vi "nanocal -- nuclear schottky fit V4.vi"() -> ()   [LabVIEW 2020] (continued)
"IDS0323_210901_RAW_cal_CeCoIn5_4th_052(138)_C(f)_12T_3.10K_45deg_Tdep_raw_.dat", "IDS0372_210908_RAW_cal_CeCoIn5_4th_102_C(f)_12.0T_3.11K_60deg_Tdep_raw_.dat", "IDS0393_210910_RAW_cal_CeCoIn5_4th_123_C(f)_8.0T_3.11K_0deg_Tdep_raw_.dat", "IDS0171_210310_RAW_cal_CeCoIn5_2nd_060_12T_fsweep_3.19K_0deg_Tdep_raw_.dat", "IDS0196_210310_RAW_cal_CeCoIn5_2nd_084_12T_5.7K_90deg_Tdep_raw_.dat", "IDS0324_210901_RAW_cal_CeCoIn5_4th_053(139)_C(f)_12T_5.70K_45deg_Tdep_raw_.dat", "IDS0373_210908_RAW_cal_CeCoIn5_4th_103_C(f)_12.0T_5.75K_60deg_Tdep_raw_.dat", "IDS0394_210910_RAW_cal_CeCoIn5_4th_124_C(f)_8.0T_5.75K_0deg_Tdep_raw_.dat", "IDS0172_210310_RAW_cal_CeCoIn5_2nd_061_12T_fsweep_5.8K_0deg_Tdep_raw_.dat"]
  in  "generate empty string from filelist !":bool
  in  "toggle generate labview files":bool
  in  "data file formatting":T13=enum."raw nanocal"
  in  "side":T14=enum."ref"
  in  "string notes":string="\"T\"-> 0.225000,    \"ζ\"-> 0.006057  , \"τ1\"-> 0.011106  , \"τS\"-> 0.134857  , \"τN\"-> 0.000042  , \"τC\"-> 0.012982  , \"κ0\"-> 0.000000101776  , \"mm1\"-> 0.000071  , \"mm2\"-> 0.148631  , \"mm3\"-> 0.011103 "
  in  "load! :l":bool
  in  "Read from file":path=path "/opt/new/Dropbox/shared_AkashAndreas/paper-CeCoIn5/Original RAW data/Original RAW files (IDS0272 to IDS03xx)/IDS0340_210904_RAW_cal_CeCoIn5_4th_069_C(f)_5.0T_0.308K_90deg_Tdep_raw_.dat"
  in  "parse! :p":bool
  in  "String":string=" <| \"ζ\"->  0.269210160049  , \"τ1\"-> 0.027533256233  , \"τS\"-> 0.109874895668  , \"τN\"-> 0.015552411517  , \"τC\"-> 0.001074349295  , \"κ0\"-> 0.000000000732  , \"mm1\"-> 0.000000000000  , \"mm2\"-> 0.000000000000  , \"mm3\"-> 0.000000000000  , \"T\"->  0.308000000000  , \"B\"-> 5.000000000000  , \"θ\"-> 90.000000000000  |> "
  out "notes":string="------------\n\n/opt/new/Dropbox/desktop_data/Indium-nanocal-cell12-June2021/labview-ready-files\nIndium_June2021_*_ark.dat\n\n---------------------\n/opt/new/Dropbox/shared_AkashAndreas/paper-CeCoIn5/labviewreadydata\nCeCoIn5_*_labview_.dat\n--------------------------------\n\n  48 ->   <| \"ζ\"->  0.219100303741  , \"τ1\"-> 0.028643012604  , \"τS\"-> 0.279362928811  , \"τN\"-> 0.246156444058  , \"τC\"-> 0.001272401549  , \"κ0\"-> 0.000000000760  , \"mm1\"-> 0.000227975653  , \"mm2\"-> 0.014929571562  , \"mm3\"-> 0.655418694024  , \"T\"->  0.148000000000  , \"B\"-> 12.000000000000  , \"θ\"-> 0.000000000000  |>   , \r49 ->   <| \"ζ\"->  0.172530402516  , \"τ1\"-> 0.028151242536  , \"τS\"-> 0.147833386881  , \"τN\"-> 0.151615465647  , \"τC\"-> 0.001078987959  , \"κ0\"-> 0.000000001040  , \"mm1\"-> 0.000157922197  , \"mm2\"-> 0.013374167913  , \"mm3\"-> 0.366811023972  , \"T\"->  0.179000000000  , \"B\"-> 12.000000000000  , \"θ\"-> 0.000000000000  |>   , \r50 ->   <| \"ζ\"->  0.133463068512  , \"τ1\"-> 0.025720252342  , \"τS\"-> 0.123146502099  , \"τN\"-> 0.097478248186  , \"τC\"-> 0.001335222055  , \"κ0\"-> 0.000000001204  , \"mm1\"-> 0.000155896243  , \"mm2\"-> 0.013755191011  , \"mm3\"-> 0.263214393590  , \"T\"->  0.197000000000  , \"B\"-> 12.000000000000  , \"θ\"-> 0.000000000000  |>   , \r51 ->   <| \"ζ\"->  0.081993362741  , \"τ1\"-> 0.028064095915  , \"τS\"-> 0.091433392476  , \"τN\"-> 0.030443971714  , \"τC\"-> 0.001450504959  , \"κ0\"-> 0.000000001536  , \"mm1\"-> 0.000108446090  , \"mm2\"-> 0.019905820843  , \"mm3\"-> 0.141370833064  , \"T\"->  0.250000000000  , \"B\"-> 12.000000000000  , \"θ\"-> 0.000000000000  |>   , \r52 ->   <| \"ζ\"->  0.054088186012  , \"τ1\"-> 0.023838802615  , \"τS\"-> 0.069079396629  , \"τN\"-> 0.016435267456  , \"τC\"-> 0.002025071743  , \"κ0\"-> 0.000000001955  , \"mm1\"-> 0.000101234646  , \"mm2\"-> 0.018244822177  , \"mm3\"-> 0.097657814678  , \"T\"->  0.300000000000  , \"B\"-> 12.000000000000  , \"θ\"-> 0.000000000000  |>   , \r53 ->   <| \"ζ\"->  0.039314966212  , \"τ1\"-> 0.020712803909  , \"τS\"-> 0.055413767550  , \"τN\"-> 0.008474403424  , \"τC\"-> 0.002674063387  , \"κ0\"-> 0.000000002415  , \"mm1\"-> 0.000096818147  , \"mm2\"-> 0.017190811405  , \"mm3\"-> 0.072499170001  , \"T\"->  0.360000000000  , \"B\"-> 12.000000000000  , \"θ\"-> 0.000000000000  |>   , \r54 ->   <| \"ζ\"->  0.031945976845  , \"τ1\"-> 0.019000922826  , \"τS\"-> 0.045624146388  , \"τN\"-> 0.005314716063  , \"τC\"-> 0.002488383471  , \"κ0\"-> 0.000000002954  , \"mm1\"-> 0.000073272643  , \"mm2\"-> 0.016306894362  , \"mm3\"-> 0.057675293464  , \"T\"->  0.430000000000  , \"B\"-> 12.000000000000  , \"θ\"-> 0.000000000000  |>   , \r55 ->   <| \"ζ\"->  0.023031239946  , \"τ1\"-> 0.018268814012  , \"τS\"-> 0.037269400776  , \"τN\"-> 0.002696792890  , \"τC\"-> 0.003257395394  , \"κ0\"-> 0.000000003720  , \"mm1\"-> 0.000067670174  , \"mm2\"-> 0.016445281937  , \"mm3\"-> 0.045899921957  , \"T\"->  0.512000000000  , \"B\"-> 12.000000000000  , \"θ\"-> 0.000000000000  |>   , \r56 ->   <| \"ζ\"->  0.019920170845  , \"τ1\"-> 0.016368892412  , \"τS\"-> 0.030579536580  , \"τN\"-> 0.001736017565  , \"τC\"-> 0.004971418152  , \"κ0\"-> 0.000000004410  , \"mm1\"-> 0.000083939556  , \"mm2\"-> 0.015095997595  , \"mm3\"-> 0.039119658918  , \"T\"->  0.610000000000  , \"B\"-> 12.000000000000  , \"θ\"-> 0.000000000000  |>   , \r57 ->   <| \"ζ\"->  0.017558473054  , \"τ1\"-> 0.014545104284  , \"τS\"-> 0.022979681288  , \"τN\"-> 0.000840829385  , \"τC\"-> 0.005228030240  , \"κ0\"-> 0.000000006068  , \"mm1\"-> 0.000073916527  , \"mm2\"-> 0.013750428362  , \"mm3\"-> 0.030187552103  , \"T\"->  0.810000000000  , \"B\"-> 12.000000000000  , \"θ\"-> 0.000000000000  |>   , \r58 ->   <| \"ζ\"->  0.011916480594  , \"τ1\"-> 0.012551282481  , \"τS\"-> 0.018233218660  , \"τN\"-> 0.000345702746  , \"τC\"-> 0.004699451527  , \"κ0\"-> 0.000000008451  , \"mm1\"-> 0.000044190864  , \"mm2\"-> 0.012162820727  , \"mm3\"-> 0.023844039179  , \"T\"->  1.120000000000  , \"B\"-> 12.000000000000  , \"θ\"-> 0.000000000000  |>   , \r59 ->   <| \"ζ\"->  0.012831327568  , \"τ1\"-> 0.013315909415  , \"τS\"-> 0.012590836847  , \"τN\"-> 0.000065003013  , \"τC\"-> 0.005276356243  , \"κ0\"-> 0.000000013610  , \"mm1\"-> 0.000047406274  , \"mm2\"-> 0.013137605540  , \"mm3\"-> 0.018225484932  , \"T\"->  1.800000000000  , \"B\"-> 12.000000000000  , \"θ\"-> 0.000000000000  |>   , \r60 ->   <| \"ζ\"->  0.019774146838  , \"τ1\"-> 0.013257273421  , \"τS\"-> 0.007064131508  , \"τN\"-> 0.000028000819  , \"τC\"-> 0.006942241845  , \"κ0\"-> 0.000000023477  , \"mm1\"-> 0.000068886863  , \"mm2\"-> 0.012935419574  , \"mm3\"-> 0.014427582022  , \"T\"->  3.000000000000  , \"B\"-> 12.000000000000  , \"θ\"-> 0.000000000000  |>   , \r61 ->   <| \"ζ\"->  0.029251354442  , \"τ1\"-> 0.014634751206  , \"τS\"-> 0.003873958746  , \"τN\"-> 0.000007000487  , \"τC\"-> 0.006827504775  , \"κ0\"-> 0.000000056438  , \"mm1\"-> 0.000072018576  , \"mm2\"-> 0.010723236476  , \"mm3\"-> 0.014661483476  , \"T\"->  5.500000000000  , \"B\"-> 12.000000000000  , \"θ\"-> 0.000000000000  |>   , \r70 ->   <| \"ζ\"->  0.166131699293  , \"τ1\"-> 0.072775930308  , \"τS\"-> 0.042465819987  , \"τN\"-> 0.161702990281  , \"τC\"-> 0.001278548133  , \"κ0\"-> 0.000000001029  , \"mm1\"-> 0.000178150965  , \"mm2\"-> 0.012296129795  , \"mm3\"-> 0.299667919341  , \"T\"->  0.179000000000  , \"B\"-> 12.000000000000  , \"θ\"-> 90.000000000000  |>   , \r71 ->   <| \"ζ\"->  0.300863384227  , \"τ1\"-> 0.104924004009  , \"τS\"-> 0.071070599729  , \"τN\"-> 0.992887187112  , \"τC\"-> 0.001721587800  , \"κ0\"-> 0.000000000548  , \"mm1\"-> 0.000392216822  , \"mm2\"-> 0.006637384427  , \"mm3\"-> 1.483679717825  , \"T\"->  0.120000000000  , \"B\"-> 12.000000000000  , \"θ\"-> 90.000000000000  |>   , \r72 ->   <| \"ζ\"->  0.222191124978  , \"τ1\"-> 0.096157808510  , \"τS\"-> 0.068016409177  , \"τN\"-> 0.365932480375  , \"τC\"-> 0.001342124138  , \"κ0\"-> 0.000000000769  , \"mm1\"-> 0.000240761160  , \"mm2\"-> 0.013184061080  , \"mm3\"-> 0.614443591912  , \"T\"->  0.148000000000  , \"B\"-> 12.000000000000  , \"θ\"-> 90.000000000000  |>   , \r73 ->   <| \"ζ\"->  0.136299067728  , \"τ1\"-> 0.070555788073  , \"τS\"-> 0.041728112583  , \"τN\"-> 0.122673380524  , \"τC\"-> 0.001576035942  , \"κ0\"-> 0.000000001215  , \"mm1\"-> 0.000183611814  , \"mm2\"-> 0.014077355758  , \"mm3\"-> 0.244680119794  , \"T\"->  0.197000000000  , \"B\"-> 12.000000000000  , \"θ\"-> 90.000000000000  |>   , \r74 ->   <| \"ζ\"->  0.083818989463  , \"τ1\"-> 0.054019568165  , \"τS\"-> 0.033709166928  , \"τN\"-> 0.048192327645  , \"τC\"-> 0.001574712191  , \"κ0\"-> 0.000000001532  , \"mm1\"-> 0.000117096712  , \"mm2\"-> 0.016005996433  , \"mm3\"-> 0.128237582295  , \"T\"->  0.249000000000  , \"B\"-> 12.000000000000  , \"θ\"-> 90.000000000000  |>   , \r75 ->   <| \"ζ\"->  0.057938569833  , \"τ1\"-> 0.045244527663  , \"τS\"-> 0.029709028064  , \"τN\"-> 0.023577376257  , \"τC\"-> 0.002006607539  , \"κ0\"-> 0.000000001948  , \"mm1\"-> 0.000103608352  , \"mm2\"-> 0.017542867394  , \"mm3\"-> 0.085978401835  , \"T\"->  0.300000000000  , \"B\"-> 12.000000000000  , \"θ\"-> 90.000000000000  |>   , \r76 ->   <| \"ζ\"->  0.044154556051  , \"τ1\"-> 0.038823125235  , \"τS\"-> 0.027069314930  , \"τN\"-> 0.013601990730  , \"τC\"-> 0.002287979276  , \"κ0\"-> 0.000000002359  , \"mm1\"-> 0.000089763345  , \"mm2\"-> 0.018083678254  , \"mm3\"-> 0.065404792018  , \"T\"->  0.360000000000  , \"B\"-> 12.000000000000  , \"θ\"-> 90.000000000000  |>   , \r77 ->   <| \"ζ\"->  0.032748569996  , \"τ1\"-> 0.031072007290  , \"τS\"-> 0.024343937548  , \"τN\"-> 0.006961654481  , \"τC\"-> 0.002967111565  , \"κ0\"-> 0.000000002964  , \"mm1\"-> 0.000084402249  , \"mm2\"-> 0.018055855929  , \"mm3\"-> 0.048229666078  , \"T\"->  0.430000000000  , \"B\"-> 12.000000000000  , \"θ\"-> 90.000000000000  |>   , \r78 ->   <| \"ζ\"->  0.027599263457  , \"τ1\"-> 0.026239105728  , \"τS\"-> 0.022370859308  , \"τN\"-> 0.003857632966  , \"τC\"-> 0.003499360499  , \"κ0\"-> 0.000000003681  , \"mm1\"-> 0.000081816106  , \"mm2\"-> 0.017901054668  , \"mm3\"-> 0.038707974796  , \"T\"->  0.512000000000  , \"B\"-> 12.000000000000  , \"θ\"-> 90.000000000000  |>   , \r79 ->   <| \"ζ\"->  0.020568815513  , \"τ1\"-> 0.023045965648  , \"τS\"-> 0.020791387386  , \"τN\"-> 0.002229171297  , \"τC\"-> 0.004427475438  , \"κ0\"-> 0.000000004398  , \"mm1\"-> 0.000074037290  , \"mm2\"-> 0.017820522459  , \"mm3\"-> 0.033072945644  , \"T\"->  0.610000000000  , \"B\"-> 12.000000000000  , \"θ\"-> 90.000000000000  |>   , \r80 ->   <| \"ζ\"->  0.016159836955  , \"τ1\"-> 0.019958638777  , \"τS\"-> 0.018730096307  , \"τN\"-> 0.000899236968  , \"τC\"-> 0.005152267403  , \"κ0\"-> 0.000000006087  , \"mm1\"-> 0.000064651231  , \"mm2\"-> 0.017530317649  , \"mm3\"-> 0.027462477400  , \"T\"->  0.810000000000  , \"B\"-> 12.000000000000  , \"θ\"-> 90.000000000000  |>   , \r81 ->   <| \"ζ\"->  0.014495870556  , \"τ1\"-> 0.019990087457  , \"τS\"-> 0.016832201384  , \"τN\"-> 0.000455517238  , \"τC\"-> 0.005555782498  , \"κ0\"-> 0.000000008420  , \"mm1\"-> 0.000060055560  , \"mm2\"-> 0.018114231010  , \"mm3\"-> 0.024909902538  , \"T\"->  1.100000000000  , \"B\"-> 12.000000000000  , \"θ\"-> 90.000000000000  |>   , \r82 ->   <| \"ζ\"->  0.014043763709  , \"τ1\"-> 0.018292068543  , \"τS\"-> 0.011311396743  , \"τN\"-> 0.000128802259  , \"τC\"-> 0.008087849636  , \"κ0\"-> 0.000000014258  , \"mm1\"-> 0.000065912054  , \"mm2\"-> 0.017276417784  , \"mm3\"-> 0.020638450794  , \"T\"->  1.800000000000  , \"B\"-> 12.000000000000  , \"θ\"-> 90.000000000000  |>   , \r83 ->   <| \"ζ\"->  0.016187684631  , \"τ1\"-> 0.018325345271  , \"τS\"-> 0.007510087776  , \"τN\"-> 0.000028419157  , \"τC\"-> 0.008115463080  , \"κ0\"-> 0.000000024747  , \"mm1\"-> 0.000062903858  , \"mm2\"-> 0.015524812312  , \"mm3\"-> 0.018513630087  , \"T\"->  3.000000000000  , \"B\"-> 12.000000000000  , \"θ\"-> 90.000000000000  |>   , \r84 ->   <| \"ζ\"->  0.027897403691  , \"τ1\"-> 0.014639690770  , \"τS\"-> 0.004105291179  , \"τN\"-> 0.000006999171  , \"τC\"-> 0.007414449545  , \"κ0\"-> 0.000000059701  , \"mm1\"-> 0.000073450671  , \"mm2\"-> 0.011534391407  , \"mm3\"-> 0.014673310811  , \"T\"->  5.700000000000  , \"B\"-> 12.000000000000  , \"θ\"-> 90.000000000000  |>   , \r"
  out "all short filenames":map{string, string}(c390)={"IDS0158_210310_RAW_cal__ref_"="IDS0158_210310_RAW_cal_CeCoIn5_2nd_047_12T_fsweep_final_0.14K_0deg_Tdep_raw_.dat", "IDS0158_210310_RAW_cal__sam_"="IDS0158_210310_RAW_cal_CeCoIn5_2nd_047_12T_fsweep_final_0.14K_0deg_Tdep_raw_.dat", "IDS0159_210310_RAW_cal__ref_"="IDS0159_210310_RAW_cal_CeCoIn5_2nd_048_12T_fsweep_0.17K_0deg_Tdep_raw_.dat", "IDS0159_210310_RAW_cal__sam_"="IDS0159_210310_RAW_cal_CeCoIn5_2nd_048_12T_fsweep_0.17K_0deg_Tdep_raw_.dat", "IDS0160_210310_RAW_cal__ref_"="IDS0160_210310_RAW_cal_CeCoIn5_2nd_049_12T_fsweep_0.20K_0deg_Tdep_raw_.dat", "IDS0160_210310_RAW_cal__sam_"="IDS0160_210310_RAW_cal_CeCoIn5_2nd_049_12T_fsweep_0.20K_0deg_Tdep_raw_.dat", "IDS0161_210310_RAW_cal__ref_"="IDS0161_210310_RAW_cal_CeCoIn5_2nd_050_12T_fsweep_0.22K_0deg_Tdep_raw_.dat", "IDS0161_210310_RAW_cal__sam_"="IDS0161_210310_RAW_cal_CeCoIn5_2nd_050_12T_fsweep_0.22K_0deg_Tdep_raw_.dat", "IDS0162_210310_RAW_cal__ref_"="IDS0162_210310_RAW_cal_CeCoIn5_2nd_051_12T_fsweep_0.28K_0deg_Tdep_raw_.dat", "IDS0162_210310_RAW_cal__sam_"="IDS0162_210310_RAW_cal_CeCoIn5_2nd_051_12T_fsweep_0.28K_0deg_Tdep_raw_.dat", "IDS0163_210310_RAW_cal__ref_"="IDS0163_210310_RAW_cal_CeCoIn5_2nd_052_12T_fsweep_0.33K_0deg_Tdep_raw_.dat", "IDS0163_210310_RAW_cal__sam_"="IDS0163_210310_RAW_cal_CeCoIn5_2nd_052_12T_fsweep_0.33K_0deg_Tdep_raw_.dat", "IDS0164_210310_RAW_cal__ref_"="IDS0164_210310_RAW_cal_CeCoIn5_2nd_053_12T_fsweep_0.40K_0deg_Tdep_raw_.dat", "IDS0164_210310_RAW_cal__sam_"="IDS0164_210310_RAW_cal_CeCoIn5_2nd_053_12T_fsweep_0.40K_0deg_Tdep_raw_.dat", "IDS0165_210310_RAW_cal__ref_"="IDS0165_210310_RAW_cal_CeCoIn5_2nd_054_12T_fsweep_0.48K_0deg_Tdep_raw_.dat", "IDS0165_210310_RAW_cal__sam_"="IDS0165_210310_RAW_cal_CeCoIn5_2nd_054_12T_fsweep_0.48K_0deg_Tdep_raw_.dat", "IDS0166_210310_RAW_cal__ref_"="IDS0166_210310_RAW_cal_CeCoIn5_2nd_055_12T_fsweep_0.58K_0deg_Tdep_raw_.dat", "IDS0166_210310_RAW_cal__sam_"="IDS0166_210310_RAW_cal_CeCoIn5_2nd_055_12T_fsweep_0.58K_0deg_Tdep_raw_.dat", "IDS0167_210310_RAW_cal__ref_"="IDS0167_210310_RAW_cal_CeCoIn5_2nd_056_12T_fsweep_0.68K_0deg_Tdep_raw_.dat", "IDS0167_210310_RAW_cal__sam_"="IDS0167_210310_RAW_cal_CeCoIn5_2nd_056_12T_fsweep_0.68K_0deg_Tdep_raw_.dat", "IDS0168_210310_RAW_cal__ref_"="IDS0168_210310_RAW_cal_CeCoIn5_2nd_057_12T_fsweep_0.91K_0deg_Tdep_raw_.dat", "IDS0168_210310_RAW_cal__sam_"="IDS0168_210310_RAW_cal_CeCoIn5_2nd_057_12T_fsweep_0.91K_0deg_Tdep_raw_.dat", "IDS0169_210310_RAW_cal__ref_"="IDS0169_210310_RAW_cal_CeCoIn5_2nd_058_12T_fsweep_1.23K_0deg_Tdep_raw_.dat", "IDS0169_210310_RAW_cal__sam_"="IDS0169_210310_RAW_cal_CeCoIn5_2nd_058_12T_fsweep_1.23K_0deg_Tdep_raw_.dat", "IDS0170_210310_RAW_cal__ref_"="IDS0170_210310_RAW_cal_CeCoIn5_2nd_059_12T_fsweep_1.97K_0deg_Tdep_raw_.dat", "IDS0170_210310_RAW_cal__sam_"="IDS0170_210310_RAW_cal_CeCoIn5_2nd_059_12T_fsweep_1.97K_0deg_Tdep_raw_.dat", "IDS0171_210310_RAW_cal__ref_"="IDS0171_210310_RAW_cal_CeCoIn5_2nd_060_12T_fsweep_3.19K_0deg_Tdep_raw_.dat", "IDS0171_210310_RAW_cal__sam_"="IDS0171_210310_RAW_cal_CeCoIn5_2nd_060_12T_fsweep_3.19K_0deg_Tdep_raw_.dat", "IDS0172_210310_RAW_cal__ref_"="IDS0172_210310_RAW_cal_CeCoIn5_2nd_061_12T_fsweep_5.8K_0deg_Tdep_raw_.dat", "IDS0172_210310_RAW_cal__sam_"="IDS0172_210310_RAW_cal_CeCoIn5_2nd_061_12T_fsweep_5.8K_0deg_Tdep_raw_.dat", "IDS0181_210310_RAW_cal__ref_"="IDS0181_210310_RAW_cal_CeCoIn5_2nd_070_12T_0.179K_90deg_fsweep_Tdep_raw_.dat", "IDS0181_210310_RAW_cal__sam_"="IDS0181_210310_RAW_cal_CeCoIn5_2nd_070_12T_0.179K_90deg_fsweep_Tdep_raw_.dat", "IDS0183_210310_RAW_cal__ref_"="IDS0183_210310_RAW_cal_CeCoIn5_2nd_071_12T_0.120K_90deg_Tdep_raw_.dat", "IDS0183_210310_RAW_cal__sam_"="IDS0183_210310_RAW_cal_CeCoIn5_2nd_071_12T_0.120K_90deg_Tdep_raw_.dat", "IDS0184_210310_RAW_cal__ref_"="IDS0184_210310_RAW_cal_CeCoIn5_2nd_072_12T_0.148K_90deg_Tdep_raw_.dat", "IDS0184_210310_RAW_cal__sam_"="IDS0184_210310_RAW_cal_CeCoIn5_2nd_072_12T_0.148K_90deg_Tdep_raw_.dat", "IDS0185_210310_RAW_cal__ref_"="IDS0185_210310_RAW_cal_CeCoIn5_2nd_073_12T_0.197K_90deg_Tdep_raw_.dat", "IDS0185_210310_RAW_cal__sam_"="IDS0185_210310_RAW_cal_CeCoIn5_2nd_073_12T_0.197K_90deg_Tdep_raw_.dat", "IDS0186_210310_RAW_cal__ref_"="IDS0186_210310_RAW_cal_CeCoIn5_2nd_074_12T_0.249K_90deg_Tdep_raw_.dat", "IDS0186_210310_RAW_cal__sam_"="IDS0186_210310_RAW_cal_CeCoIn5_2nd_074_12T_0.249K_90deg_Tdep_raw_.dat", "IDS0187_210310_RAW_cal__ref_"="IDS0187_210310_RAW_cal_CeCoIn5_2nd_075_12T_0.300K_90deg_Tdep_raw_.dat", "IDS0187_210310_RAW_cal__sam_"="IDS0187_210310_RAW_cal_CeCoIn5_2nd_075_12T_0.300K_90deg_Tdep_raw_.dat", "IDS0188_210310_RAW_cal__ref_"="IDS0188_210310_RAW_cal_CeCoIn5_2nd_076_12T_0.360K_90deg_Tdep_raw_.dat", "IDS0188_210310_RAW_cal__sam_"="IDS0188_210310_RAW_cal_CeCoIn5_2nd_076_12T_0.360K_90deg_Tdep_raw_.dat", "IDS0189_210310_RAW_cal__ref_"="IDS0189_210310_RAW_cal_CeCoIn5_2nd_077_12T_0.430K_90deg_Tdep_raw_.dat", "IDS0189_210310_RAW_cal__sam_"="IDS0189_210310_RAW_cal_CeCoIn5_2nd_077_12T_0.430K_90deg_Tdep_raw_.dat", "IDS0190_210310_RAW_cal__ref_"="IDS0190_210310_RAW_cal_CeCoIn5_2nd_078_12T_0.512K_90deg_Tdep_raw_.dat", "IDS0190_210310_RAW_cal__sam_"="IDS0190_210310_RAW_cal_CeCoIn5_2nd_078_12T_0.512K_90deg_Tdep_raw_.dat", "IDS0191_210310_RAW_cal__ref_"="IDS0191_210310_RAW_cal_CeCoIn5_2nd_079_12T_0.610K_90deg_Tdep_raw_.dat", "IDS0191_210310_RAW_cal__sam_"="IDS0191_210310_RAW_cal_CeCoIn5_2nd_079_12T_0.610K_90deg_Tdep_raw_.dat", "IDS0192_210310_RAW_cal__ref_"="IDS0192_210310_RAW_cal_CeCoIn5_2nd_080_12T_0.810K_90deg_Tdep_raw_.dat", "IDS0192_210310_RAW_cal__sam_"="IDS0192_210310_RAW_cal_CeCoIn5_2nd_080_12T_0.810K_90deg_Tdep_raw_.dat", "IDS0193_210310_RAW_cal__ref_"="IDS0193_210310_RAW_cal_CeCoIn5_2nd_081_12T_1.1K_90deg_Tdep_raw_.dat", "IDS0193_210310_RAW_cal__sam_"="IDS0193_210310_RAW_cal_CeCoIn5_2nd_081_12T_1.1K_90deg_Tdep_raw_.dat", "IDS0194_210310_RAW_cal__ref_"="IDS0194_210310_RAW_cal_CeCoIn5_2nd_082_12T_1.8K_90deg_Tdep_raw_.dat", "IDS0194_210310_RAW_cal__sam_"="IDS0194_210310_RAW_cal_CeCoIn5_2nd_082_12T_1.8K_90deg_Tdep_raw_.dat", "IDS0195_210310_RAW_cal__ref_"="IDS0195_210310_RAW_cal_CeCoIn5_2nd_083_12T_3.0K_90deg_Tdep_raw_.dat", "IDS0195_210310_RAW_cal__sam_"="IDS0195_210310_RAW_cal_CeCoIn5_2nd_083_12T_3.0K_90deg_Tdep_raw_.dat", "IDS0196_210310_RAW_cal__ref_"="IDS0196_210310_RAW_cal_CeCoIn5_2nd_084_12T_5.7K_90deg_Tdep_raw_.dat", "IDS0196_210310_RAW_cal__sam_"="IDS0196_210310_RAW_cal_CeCoIn5_2nd_084_12T_5.7K_90deg_Tdep_raw_.dat", "IDS0208_210310_RAW_cal__ref_"="IDS0208_210310_RAW_cal_CeCoIn5_2nd_096_Hsweep_0.197K_Tdep_raw_.dat", "IDS0208_210310_RAW_cal__sam_"="IDS0208_210310_RAW_cal_CeCoIn5_2nd_096_Hsweep_0.197K_Tdep_raw_.dat", "IDS0209_210310_RAW_cal__ref_"="IDS0209_210310_RAW_cal_CeCoIn5_2nd_097_Hsweep_0.197K_Tdep_raw_.dat", "IDS0209_210310_RAW_cal__sam_"="IDS0209_210310_RAW_cal_CeCoIn5_2nd_097_Hsweep_0.197K_Tdep_raw_.dat", "IDS0210_210310_RAW_cal__ref_"="IDS0210_210310_RAW_cal_CeCoIn5_2nd_098_fsweep_6T_0.148K_Bdep_raw_.dat", "IDS0210_210310_RAW_cal__sam_"="IDS0210_210310_RAW_cal_CeCoIn5_2nd_098_fsweep_6T_0.148K_Bdep_raw_.dat", "IDS0211_210310_RAW_cal__ref_"="IDS0211_210310_RAW_cal_CeCoIn5_2nd_099_fsweep_9T_0.197K_Bdep_raw_.dat", "IDS0211_210310_RAW_cal__sam_"="IDS0211_210310_RAW_cal_CeCoIn5_2nd_099_fsweep_9T_0.197K_Bdep_raw_.dat", "IDS0212_210310_RAW_cal__ref_"="IDS0212_210310_RAW_cal_CeCoIn5_2nd_100_fsweep_11T_0.197K_Bdep_raw_.dat", "IDS0212_210310_RAW_cal__sam_"="IDS0212_210310_RAW_cal_CeCoIn5_2nd_100_fsweep_11T_0.197K_Bdep_raw_.dat", "IDS0213_210310_RAW_cal__ref_"="IDS0213_210310_RAW_cal_CeCoIn5_2nd_101_fsweep_10T_0.197K_Bdep_raw_.dat", "IDS0213_210310_RAW_cal__sam_"="IDS0213_210310_RAW_cal_CeCoIn5_2nd_101_fsweep_10T_0.197K_Bdep_raw_.dat", "IDS0214_210310_RAW_cal__ref_"="IDS0214_210310_RAW_cal_CeCoIn5_2nd_102_fsweep_8T_0.197K_Bdep_raw_.dat", "IDS0214_210310_RAW_cal__sam_"="IDS0214_210310_RAW_cal_CeCoIn5_2nd_102_fsweep_8T_0.197K_Bdep_raw_.dat", "IDS0215_210310_RAW_cal__ref_"="IDS0215_210310_RAW_cal_CeCoIn5_2nd_103_fsweep_7T_0.197K_Bdep_raw_.dat", "IDS0215_210310_RAW_cal__sam_"="IDS0215_210310_RAW_cal_CeCoIn5_2nd_103_fsweep_7T_0.197K_Bdep_raw_.dat", "IDS0216_210310_RAW_cal__ref_"="IDS0216_210310_RAW_cal_CeCoIn5_2nd_104_fsweep_5T_0.197K_Bdep_raw_.dat", "IDS0216_210310_RAW_cal__sam_"="IDS0216_210310_RAW_cal_CeCoIn5_2nd_104_fsweep_5T_0.197K_Bdep_raw_.dat", "IDS0217_210310_RAW_cal__ref_"="IDS0217_210310_RAW_cal_CeCoIn5_2nd_105_fsweep_0T_0.197K_Bdep_raw_.dat", "IDS0217_210310_RAW_cal__sam_"="IDS0217_210310_RAW_cal_CeCoIn5_2nd_105_fsweep_0T_0.197K_Bdep_raw_.dat", "IDS0218_210310_RAW_cal__ref_"="IDS0218_210310_RAW_cal_CeCoIn5_2nd_106_fsweep_0T_1.55K_Bdep_raw_.dat", "IDS0218_210310_RAW_cal__sam_"="IDS0218_210310_RAW_cal_CeCoIn5_2nd_106_fsweep_0T_1.55K_Bdep_raw_.dat", "IDS0219_210310_RAW_cal__ref_"="IDS0219_210310_RAW_cal_CeCoIn5_2nd_107_fsweep_0T_1.0K_Bdep_raw_.dat", "IDS0219_210310_RAW_cal__sam_"="IDS0219_210310_RAW_cal_CeCoIn5_2nd_107_fsweep_0T_1.0K_Bdep_raw_.dat", "IDS0220_210310_RAW_cal__ref_"="IDS0220_210310_RAW_cal_CeCoIn5_2nd_108_fsweep_0T_0.677K_Bdep_raw_.dat", "IDS0220_210310_RAW_cal__sam_"="IDS0220_210310_RAW_cal_CeCoIn5_2nd_108_fsweep_0T_0.677K_Bdep_raw_.dat", "IDS0293_210427_RAW_cal__ref_"="IDS0293_210427_RAW_cal_CeCoIn5_4th_022(123)_C(f)_12T_1.90K_30deg_NEW_Tdep_raw_.dat", "IDS0293_210427_RAW_cal__sam_"="IDS0293_210427_RAW_cal_CeCoIn5_4th_022(123)_C(f)_12T_1.90K_30deg_NEW_Tdep_raw_.dat", "IDS0294_210427_RAW_cal__ref_"="IDS0294_210427_RAW_cal_CeCoIn5_4th_023(122)_C(f)_12T_1.13K_30deg_NEW_Tdep_raw_.dat", "IDS0294_210427_RAW_cal__sam_"="IDS0294_210427_RAW_cal_CeCoIn5_4th_023(122)_C(f)_12T_1.13K_30deg_NEW_Tdep_raw_.dat", "IDS0295_210427_RAW_cal__ref_"="IDS0295_210427_RAW_cal_CeCoIn5_4th_024(121)_C(f)_12T_0.83K_30deg_NEW_Tdep_raw_.dat", "IDS0295_210427_RAW_cal__sam_"="IDS0295_210427_RAW_cal_CeCoIn5_4th_024(121)_C(f)_12T_0.83K_30deg_NEW_Tdep_raw_.dat", "IDS0296_210427_RAW_cal__ref_"="IDS0296_210427_RAW_cal_CeCoIn5_4th_025(120)_C(f)_12T_0.62K_30deg_NEW_Tdep_raw_.dat", "IDS0296_210427_RAW_cal__sam_"="IDS0296_210427_RAW_cal_CeCoIn5_4th_025(120)_C(f)_12T_0.62K_30deg_NEW_Tdep_raw_.dat", "IDS0297_210427_RAW_cal__ref_"="IDS0297_210427_RAW_cal_CeCoIn5_4th_026(119)_C(f)_12T_0.53K_30deg_NEW_Tdep_raw_.dat", "IDS0297_210427_RAW_cal__sam_"="IDS0297_210427_RAW_cal_CeCoIn5_4th_026(119)_C(f)_12T_0.53K_30deg_NEW_Tdep_raw_.dat", "IDS0298_210427_RAW_cal__ref_"="IDS0298_210427_RAW_cal_CeCoIn5_4th_027(118)_C(f)_12T_0.43K_30deg_NEW_Tdep_raw_.dat", "IDS0298_210427_RAW_cal__sam_"="IDS0298_210427_RAW_cal_CeCoIn5_4th_027(118)_C(f)_12T_0.43K_30deg_NEW_Tdep_raw_.dat", "IDS0299_210427_RAW_cal__ref_"="IDS0299_210427_RAW_cal_CeCoIn5_4th_028(117)_C(f)_12T_0.36K_30deg_NEW_Tdep_raw_.dat", "IDS0299_210427_RAW_cal__sam_"="IDS0299_210427_RAW_cal_CeCoIn5_4th_028(117)_C(f)_12T_0.36K_30deg_NEW_Tdep_raw_.dat", "IDS0300_210427_RAW_cal__ref_"="IDS0300_210427_RAW_cal_CeCoIn5_4th_029(113)_C(f)_12T_0.14K_30deg_NEW_Tdep_raw_.dat", "IDS0300_210427_RAW_cal__sam_"="IDS0300_210427_RAW_cal_CeCoIn5_4th_029(113)_C(f)_12T_0.14K_30deg_NEW_Tdep_raw_.dat", "IDS0301_210831_RAW_cal__ref_"="IDS0301_210831_RAW_cal_CeCoIn5_4th_030(116)_C(f)_12T_0.30K_30deg_NEW_Tdep_raw_.dat", "IDS0301_210831_RAW_cal__sam_"="IDS0301_210831_RAW_cal_CeCoIn5_4th_030(116)_C(f)_12T_0.30K_30deg_NEW_Tdep_raw_.dat", "IDS0302_210831_RAW_cal__ref_"="IDS0302_210831_RAW_cal_CeCoIn5_4th_031(115)_C(f)_12T_0.25K_30deg_NEW_Tdep_raw_.dat", "IDS0302_210831_RAW_cal__sam_"="IDS0302_210831_RAW_cal_CeCoIn5_4th_031(115)_C(f)_12T_0.25K_30deg_NEW_Tdep_raw_.dat", "IDS0303_210831_RAW_cal__ref_"="IDS0303_210831_RAW_cal_CeCoIn5_4th_032(114)_C(f)_12T_0.20K_30deg_NEW_Tdep_raw_.dat", "IDS0303_210831_RAW_cal__sam_"="IDS0303_210831_RAW_cal_CeCoIn5_4th_032(114)_C(f)_12T_0.20K_30deg_NEW_Tdep_raw_.dat", "IDS0304_210831_RAW_cal__ref_"="IDS0304_210831_RAW_cal_CeCoIn5_4th_033(112)_C(f)_12T_0.17K_30deg_NEW_Tdep_raw_.dat", "IDS0304_210831_RAW_cal__sam_"="IDS0304_210831_RAW_cal_CeCoIn5_4th_033(112)_C(f)_12T_0.17K_30deg_NEW_Tdep_raw_.dat", "IDS0305_210831_RAW_cal__ref_"="IDS0305_210831_RAW_cal_CeCoIn5_4th_034(110)_C(f)_12T_0.16K_30deg_NEW_Tdep_raw_.dat", "IDS0305_210831_RAW_cal__sam_"="IDS0305_210831_RAW_cal_CeCoIn5_4th_034(110)_C(f)_12T_0.16K_30deg_NEW_Tdep_raw_.dat", "IDS0306_210831_RAW_cal__ref_"="IDS0306_210831_RAW_cal_CeCoIn5_4th_035(124)_C(f)_12T_3.10K_30deg_NEW_Tdep_raw_.dat", "IDS0306_210831_RAW_cal__sam_"="IDS0306_210831_RAW_cal_CeCoIn5_4th_035(124)_C(f)_12T_3.10K_30deg_NEW_Tdep_raw_.dat", "IDS0310_210901_RAW_cal__ref_"="IDS0310_210901_RAW_cal_CeCoIn5_4th_039(125)_C(f)_12T_0.157K_45deg_Tdep_raw_.dat", "IDS0310_210901_RAW_cal__sam_"="IDS0310_210901_RAW_cal_CeCoIn5_4th_039(125)_C(f)_12T_0.157K_45deg_Tdep_raw_.dat", "IDS0311_210901_RAW_cal__ref_"="IDS0311_210901_RAW_cal_CeCoIn5_4th_040(126)_C(f)_12T_0.120K_45deg_Tdep_raw_.dat", "IDS0311_210901_RAW_cal__sam_"="IDS0311_210901_RAW_cal_CeCoIn5_4th_040(126)_C(f)_12T_0.120K_45deg_Tdep_raw_.dat", "IDS0312_210901_RAW_cal__ref_"="IDS0312_210901_RAW_cal_CeCoIn5_4th_041(127)_C(f)_12T_0.170K_45deg_Tdep_raw_.dat", "IDS0312_210901_RAW_cal__sam_"="IDS0312_210901_RAW_cal_CeCoIn5_4th_041(127)_C(f)_12T_0.170K_45deg_Tdep_raw_.dat", "IDS0313_210901_RAW_cal__ref_"="IDS0313_210901_RAW_cal_CeCoIn5_4th_042(128)_C(f)_12T_0.200K_45deg_Tdep_raw_.dat", "IDS0313_210901_RAW_cal__sam_"="IDS0313_210901_RAW_cal_CeCoIn5_4th_042(128)_C(f)_12T_0.200K_45deg_Tdep_raw_.dat", "IDS0314_210901_RAW_cal__ref_"="IDS0314_210901_RAW_cal_CeCoIn5_4th_043(129)_C(f)_12T_0.255K_45deg_Tdep_raw_.dat", "IDS0314_210901_RAW_cal__sam_"="IDS0314_210901_RAW_cal_CeCoIn5_4th_043(129)_C(f)_12T_0.255K_45deg_Tdep_raw_.dat", "IDS0315_210901_RAW_cal__ref_"="IDS0315_210901_RAW_cal_CeCoIn5_4th_044(130)_C(f)_12T_0.300K_45deg_Tdep_raw_.dat", "IDS0315_210901_RAW_cal__sam_"="IDS0315_210901_RAW_cal_CeCoIn5_4th_044(130)_C(f)_12T_0.300K_45deg_Tdep_raw_.dat", "IDS0316_210901_RAW_cal__ref_"="IDS0316_210901_RAW_cal_CeCoIn5_4th_045(131)_C(f)_12T_0.360K_45deg_Tdep_raw_.dat", "IDS0316_210901_RAW_cal__sam_"="IDS0316_210901_RAW_cal_CeCoIn5_4th_045(131)_C(f)_12T_0.360K_45deg_Tdep_raw_.dat", "IDS0317_210901_
